vi "Auto_Inspection Station Main.vi"(8 "站別":refnum<vi>, 9 "站別":i32, 10 "ActRef":refnum<vi>, 11 "Station Action.lvclass":refnum<class "Station Action.lvclass">) -> ()   [LabVIEW 2019]
uses:
  Station Class/Station Action.lvclass
  Ctrl/Station Action.ctl
  Ctrl/Auto Inspection Data Name.ctl
  FlowCtrl Class/BarcodeScan/Ctl/Board Scan IO.ctl
  FlowCtrl Class/Ctrl/Auto Inspection_IN Name2.ctl
  Ctrl/ModbusCmd.ctl
  Ctrl/S2 Station IO.ctl
  FlowCtrl Class/Laser Detect/Ctl/S11 Station IO.ctl
  Function/Main UI/Glb/Main_UI Gb.vi
  Global/Process Global.vi
  Ctrl/Auto Inspection Main UI Ref.ctl
  LLB/Commonly VI.lvlib
  Ctrl/Auto Inspection Station Name2.ctl
  LLB/Commonly VI/Main Glb.vi
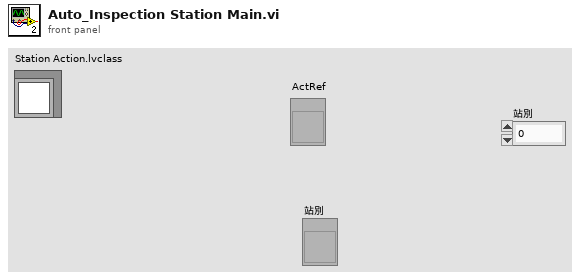
[diagram p1: front panel]
types:
  T1 = typedef "Station Action.ctl" = enum16{"Wait Item In", "Dectect Action", "ImformOut"}
  T2 = cluster{"AutoRunFlg":refnum<vi>, "Action Finish Flg":refnum<vi>, "Remaining Action":refnum<vi>, "Btn_AutoRun":refnum<vi>, "Manual Flg":refnum<vi>, "Sub Process Error":refnum<vi>}
  T3 = typedef "Auto Inspection Data Name.ctl" = enum16{"LocalRun", "ItemSN(TimeCode)", "CurrentAction", "Error", "Data", "OKNG", "電壓值", "電壓值判斷", "電流值", "電流值判斷", "Laser1 Data", "Laser2 Data", "Laser OKNG", "StationNO"}
  T4 = cluster{"starting address":u16, "number of inputs":u16, "Sat Coils":bool[], "Holding Registers":u16[]}
  T5 = typedef "ModbusCmd.ctl" = enum16{"Connect", "Disconnect", "Init", "Fetch Basic Objects", "Fetch Input Refisters", "Fetch Discrete Inputs", "Set Coils", "Set Holding Registers", "Write Single Holding", "Exit"}
  T6 = typedef "Auto Inspection_IN Name2.ctl" = enum16{"S0 Station", "S1 Barcode ", "S2 Tool Format", "S3 Tool Prpgram", "S4 Tool Sacn", "S11 Laser Detect", "S8 Vision AI"}
  T7 = typedef "Board Scan IO.ctl" = enum16{"S1 Barcode Scan", "回給PLC完成讀取訊號", "S1 載盤條碼比對NG", "S1PLC 條碼可讀取訊號", "S1備用_04", "S1備用_05", "S1備用_06", "S1備用_07", "S1備用_08", "S1 發送條碼完成"}
  T8 = typedef "S2 Station IO.ctl" = enum16{"S2站PC動作中_20", "電流量測完成產品OK_21", "電流量測完成產品NG_22", "S2站Format 執行_23", "S2 Format OK_24", "S2 Format NG_25", "S2站燒入執行_26", "S2站燒入OK_27", "S2站燒入NG_28", "S2站動作完成_29", "S3 PC動作中_30", "S3 Format 此站執行_31", "S3 Format OK_32", "S3 Format NG_33", "S3 燒入程式 此站執行_34", "S3 燒入程式 OK_35", "S3 燒入程式 NG_36", "S3 備用_37", "S3 備用_38", "S3 動作完成_39", "S4 PC動作中_40", "S4 量測完成 產品正常_41", "S4 量測完成 產品NG_42", "S4 Format 此站執行_43", "S4 Format OK_44", "S4 Format NG_45", "S4 燒入 此站不執行_46", "S4 燒入程式 OK_47", "S4 燒入程式 NG_48", "S4 藍芽Scan OK_49", "S4 藍芽Scan NG_50", "S4 動作完成_51", "給PLC要量電流訊號", "給PLC要量電壓訊號"}
  T9 = typedef "S11 Station IO.ctl" = enum16{"S11雷射測量動作中", "S11雷射測點1完成", "S11雷射測點2完成", "S11雷測測量OK", "S11雷測測量NG", "S11雷測測量重測", "S11備用_6", "S11備用_7", "S11備用_8", "S11雷射測高完成"}
  T10 = typedef "Auto Inspection Station Name2.ctl" = enum16{"S1Barcode", "S2Measure", "S3Measure", "S4Measure", "S5Measure", "S11_LaserCheck", "S8_Vision AI"}
  T11 = typedef "Auto Inspection Main UI Ref.ctl" = cluster{"LineScan arrive":refnum<vi>, "LineScanfinish":refnum<vi>, "AI arrive":refnum<vi>, "AI finish":refnum<vi>, "NG Pick arrive":refnum<vi>, "NG Pick finish":refnum<vi>}
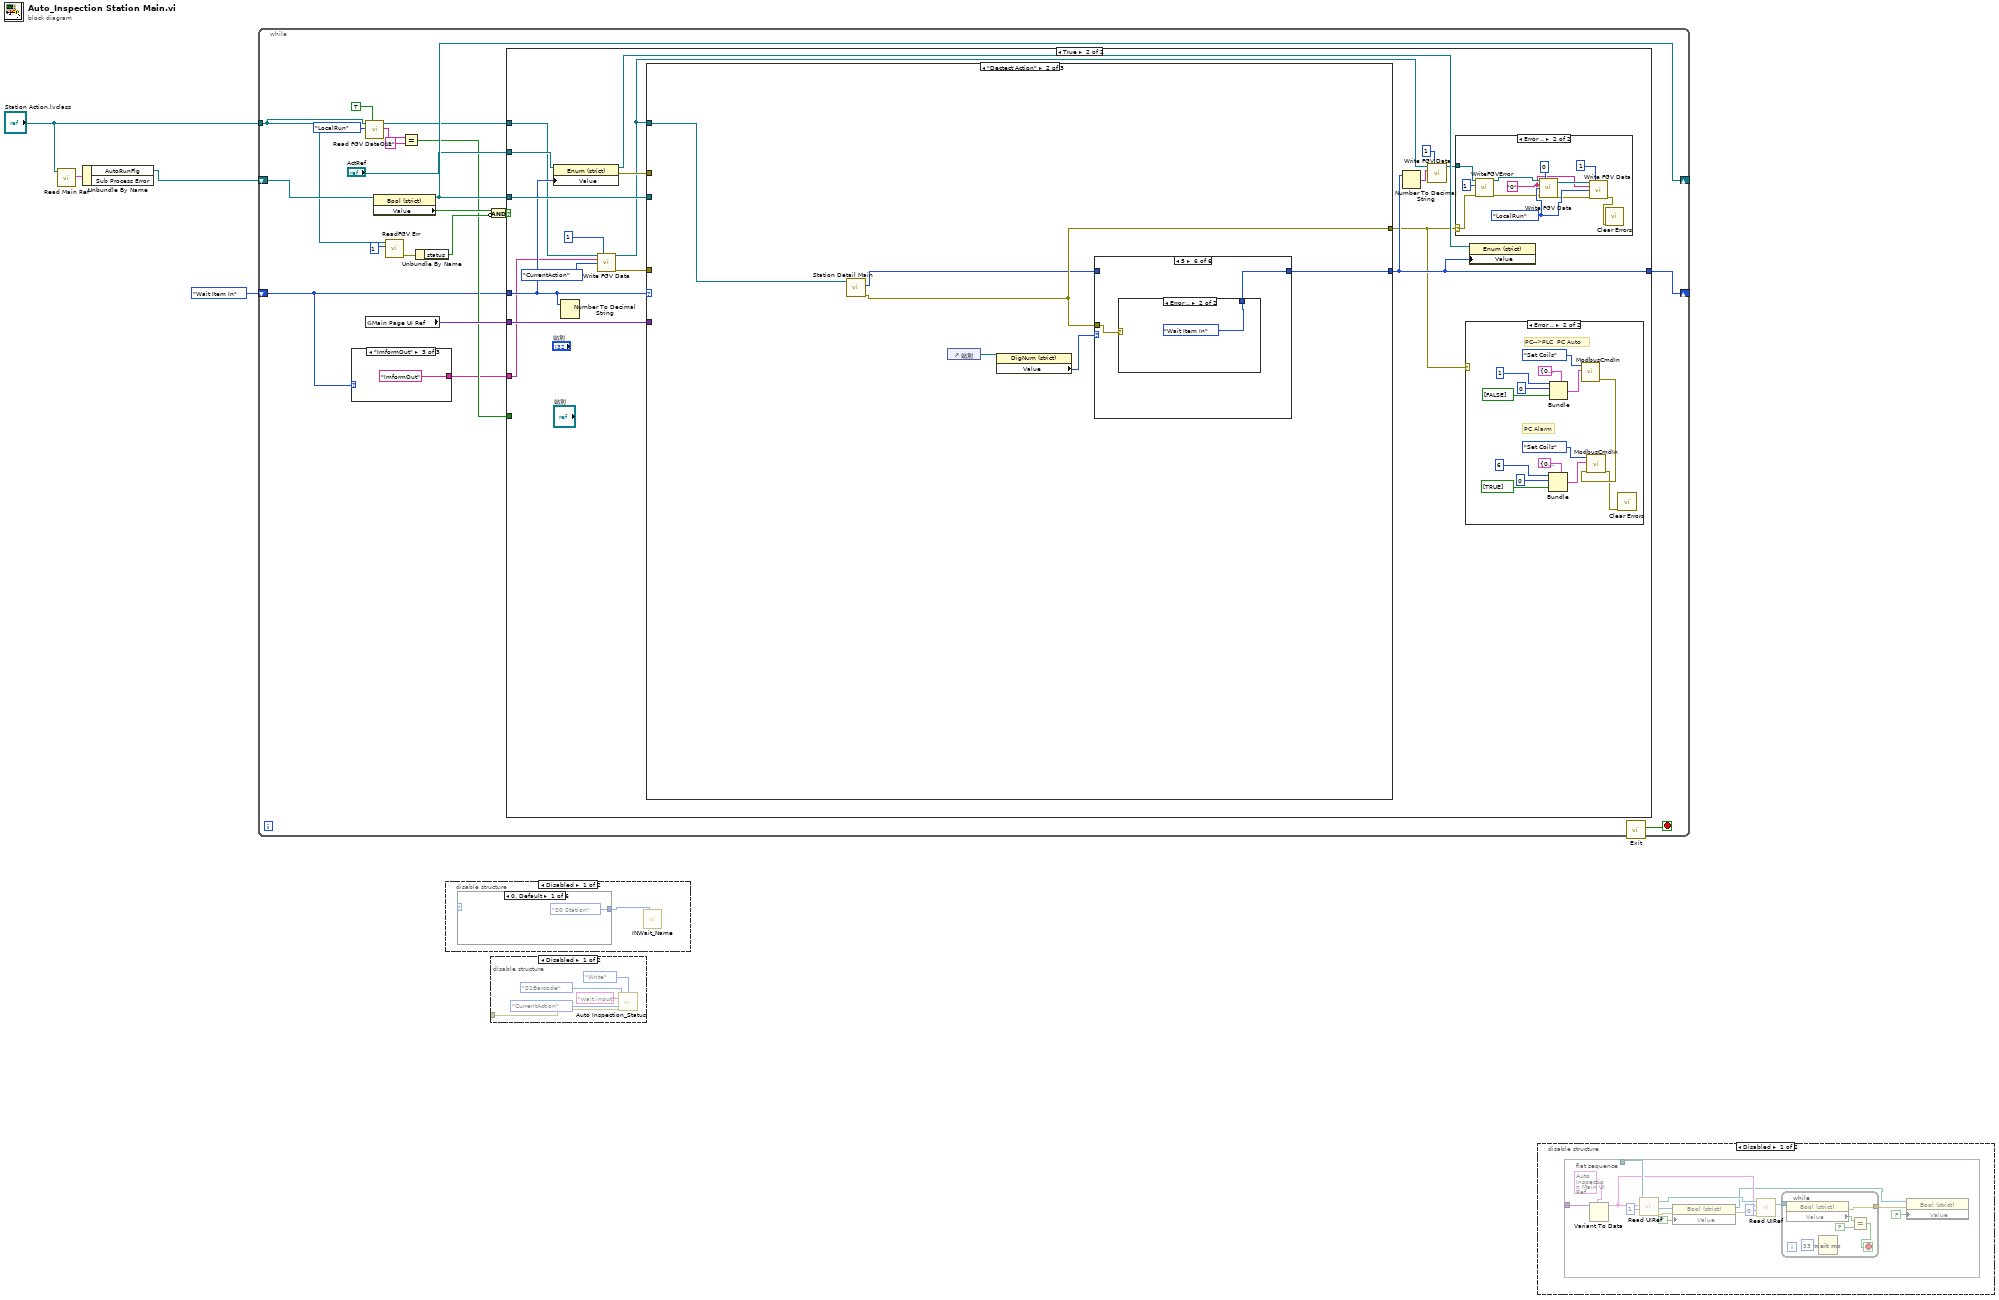
[diagram p0: block diagram]
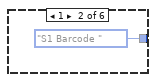
[diagram p2: hidden frame]
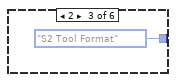
[diagram p3: hidden frame]
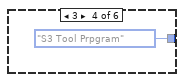
[diagram p4: hidden frame]
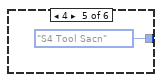
[diagram p5: hidden frame]
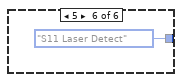
[diagram p6: hidden frame]
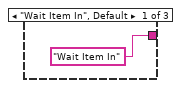
[diagram p10: hidden frame]
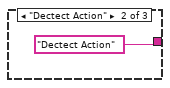
[diagram p11: hidden frame]
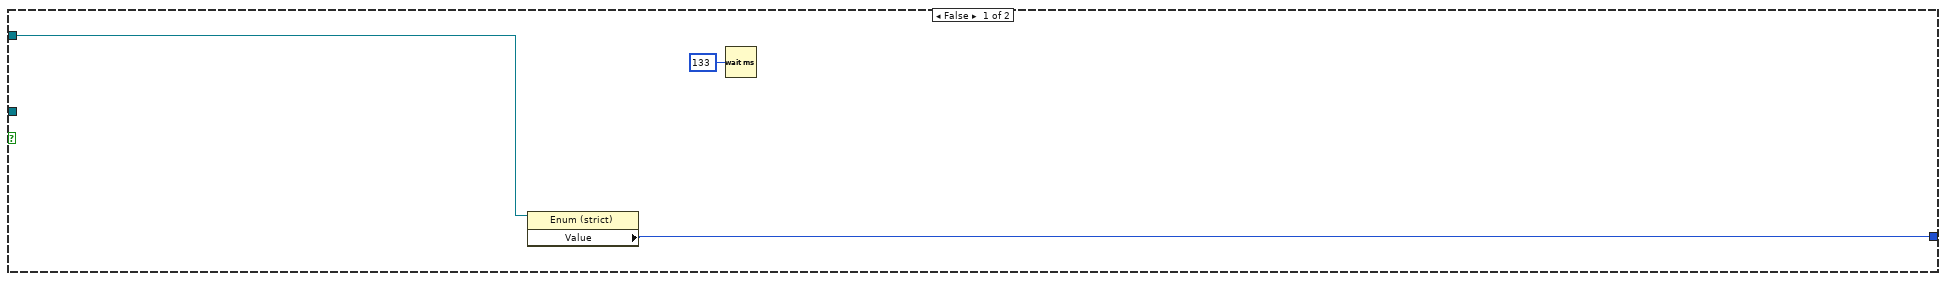
[diagram p12: hidden frame]
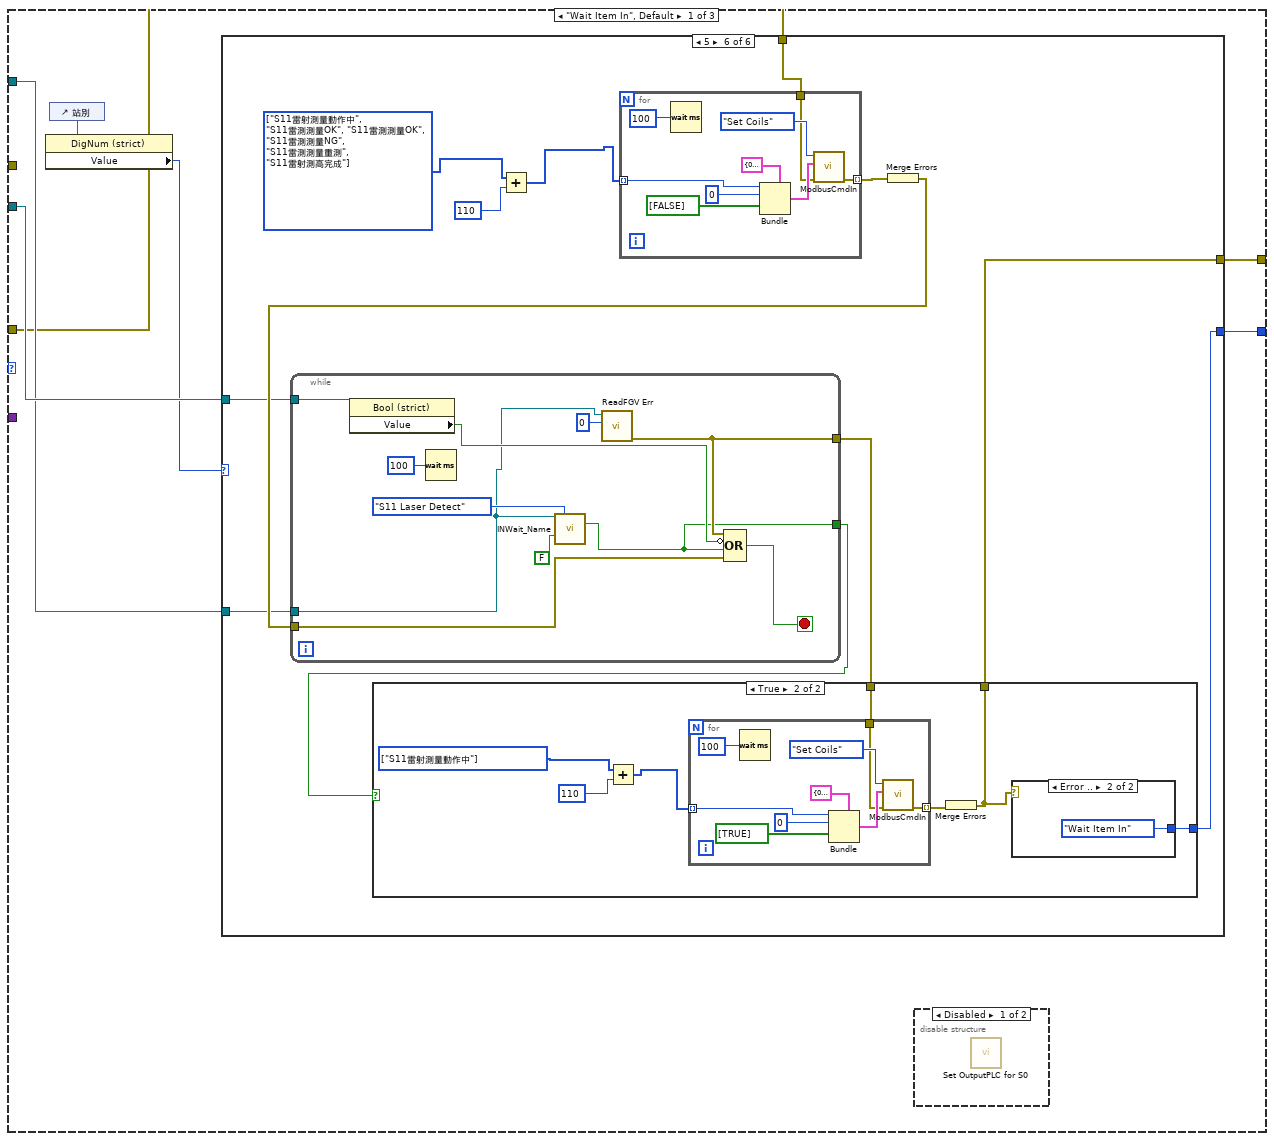
[diagram p15: hidden frame]
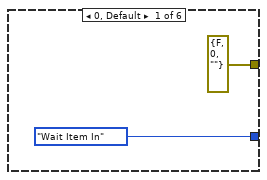
[diagram p17: hidden frame]
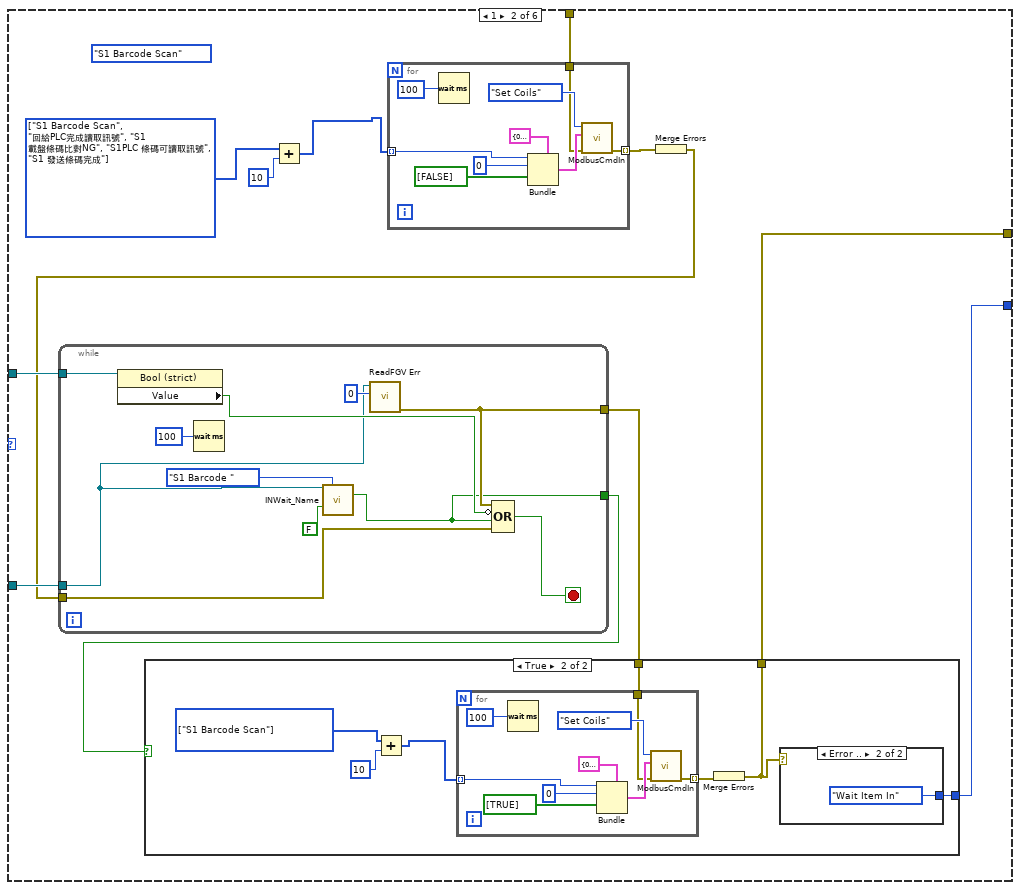
[diagram p18: hidden frame]
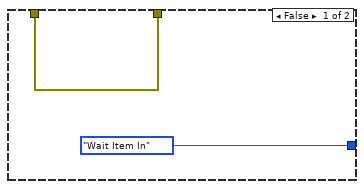
[diagram p19: hidden frame]
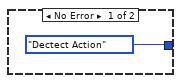
[diagram p20: hidden frame]
diagram:
  n1 = call-dynamic "Read Main Ref.vi"("Main Process Class in"="Station Action.lvclass") -> ("Main Ref"=w3:T2)  [unwired: 8 in, 2 out]
  n2 = Unbundle By Name(w3) -> ("AutoRunFlg"=w1:refnum<vi>)  [unwired: 1 out]
  n3 = while {
    shift-right: [w20] -> _
    shift-left: Station_Action."Wait Item In" -> [w6]
    tunnel: "Station Action.lvclass" -> [w8]
    shift-right: [w18] -> _
    shift-left: w1 -> [w23]
    stop <- w19 stop-if-true
    n4 = case shown="\"ImformOut\"" w6 {
      tunnel: ["Wait Item In" "Dectect Action" "ImformOut"] -> w5
      frame "Wait Item In", Default {
      }
      frame "Dectect Action" {
      }
      frame "ImformOut" {
      }
    }
    n5 = call-dynamic "Read FGV DataOut.vi"("TSt/FConveyor"=TRUE, "Data"=Auto_Inspection_Data_Name."LocalRun", "Station Action in"=w8) -> ("DataOut"=w11:string, "Station Action out"=w14:refnum<class "Station Action.lvclass">)  [unwired: 6 in, 1 out]
    n6 = global read "Main_UI Gb.vi" "Main Page UI Ref"() -> (w21:variant)
    n7 = property class="Bool (strict)"(reference=w23) -> (reference out=w18:refnum<vi>, "Value"=w24:bool)  [unwired: 1 in, 1 out]
    n8 = call-dynamic "ReadFGV Err.vi"("0Cv/1ST"=1, "Station Action in"=w8) -> ("error out"=w16:errorcluster)  [unwired: 8 in, 1 out]
    n9 = Equal?(x=w11, y="1") -> (x = y?=w7:bool)
    n10 = Unbundle By Name(w16) -> ("status"=w15:bool)
    n11 = Compound Arithmetic op=AND(w24, invert w15) -> (w22:bool)
    n12 = case shown="True" w22 {
      tunnel: w18 -> [_ w46]
      tunnel: w6 -> [_ w39]
      tunnel: w21 -> [_ w47]
      tunnel: w14 -> [_ w32]
      tunnel: [w29 w36] -> w20
      tunnel: "ActRef" -> [w30 w45]
      tunnel: w7 -> [_ _]
      tunnel: w5 -> [_ w31]
      frame False {
        n13 = property class="Enum (strict)"(reference=w30) -> ("Value"=w29:T1)  [unwired: 1 in, 2 out]
        n14 = Wait (ms)(milliseconds to wait=u32 133) -> ()  [unwired: 1 out]
      }
      frame True {
        n15 = property class="Enum (strict)"(reference=w45, "Value"=w39) -> (reference out=w44:refnum<vi>, error out=w43:errorcluster)  [unwired: 1 in]
        n16 = Number To Decimal String(number=w39) -> ()  [unwired: 1 in, 1 out]
        n17 = call-dynamic "Write FGV Data.vi"("Station Action in"=w32, "0Cv/1St"=1, "DataIn"=w31, "Data"=Auto_Inspection_Data_Name."CurrentAction") -> ("Station Action out"=w35:refnum<class "Station Action.lvclass">, "error out"=w40:errorcluster)  [unwired: 10 in]
        n18 = case shown="\"Dectect Action\"" w39 {
          tunnel: w47 -> [_ _ _]
          tunnel: w35 -> [w79 w352 w380]
          tunnel: w46 -> [w80 _ w379]
          tunnel: [w75 w350 w375] -> w36
          tunnel: w43 -> [_ _ _]
          tunnel: [w78 w351 w376] -> w33
          tunnel: w40 -> [w74 _ w378]
          frame "Wait Item In", Default {
            n19 = control-ref of="站別"() -> (w77:refnum<vi>)
            n20 = property class="DigNum (strict)"(reference=w77) -> ("Value"=w76:i32)  [unwired: 1 in, 2 out]
            n21 = case shown="5" w76 {
              tunnel: w80 -> [_ w94 w142 w195 w247 w298]
              tunnel: w79 -> [_ w93 w143 w194 w246 w300]
              tunnel: [errorcluster {"status"=FALSE, "code"=0, "source"=""} ("error IO") w92 w135 w197 w243 w299] -> w78
              tunnel: w74 -> [_ w91 _ w190 w248 w301]
              tunnel: [Station_Action."Wait Item In" w87 w144 w196 w245 w296] -> w75
              frame 0, Default {
              }
              frame 1 {
                (unwired) Board_Scan_IO."S1 Barcode Scan" ("Enum")
                w85 = T7[] [enum."S1 Barcode Scan", enum."回給PLC完成讀取訊號", enum."S1 載盤條碼比對NG", enum."S1PLC 條碼可讀取訊號", enum."S1 發送條碼完成"] items=["S1 Barcode Scan", "回給PLC完成讀取訊號", "S1 載盤條碼比對NG", "S1PLC 條碼可讀取訊號", "S1備用_04", "S1備用_05", "S1備用_06", "S1備用_07", "S1備用_08", "S1 發送條碼完成"]
                n22 = Add(x=w85, y=10) -> (x+y=w84:i32[])
                n23 = for {
                  tunnel: [w128] -> w90 mode=indexing
                  tunnel: w84 -> [w127] mode=indexing
                  tunnel: w91 -> [w126]
                  n24 = Wait (ms)(milliseconds to wait=100) -> ()  [unwired: 1 out]
                  n25 = Bundle(cluster=T4 {"starting address"=0, "number of inputs"=0, "Sat Coils"=[], "Holding Registers"=[]} ("data"), "starting address"=w127, "number of inputs"=u16 0, "Sat Coils"=bool[] [FALSE]) -> (w131:T4)  [unwired: 1 in]
                  n26 = call "ModbusCmdIn.vi"("error in (no error)"=w126, "data"=w131, "Enum"=ModbusCmd."Set Coils") -> ("error out"=w128:errorcluster)  [unwired: 8 in]
                }
                n27 = Merge Errors(w90) -> (w89:errorcluster)
                n28 = while {
                  tunnel: w94 -> [w125]
                  tunnel: w93 -> [w119]
                  tunnel: [w120] -> w88
                  tunnel: w89 -> [w117]
                  tunnel: [w116] -> w83
                  stop <- w124 stop-if-true
                  n29 = property class="Bool (strict)"(reference=w125) -> ("Value"=w122:bool)  [unwired: 1 in, 2 out]
                  n30 = Wait (ms)(milliseconds to wait=u32 100) -> ()  [unwired: 1 out]
                  n31 = call "INWait_Name.vi"("FlowCtrl in"=w119, "Input2"=Auto_Inspection_IN_Name2."S1 Barcode ", "Wait?"=FALSE) -> ("StatusOut"=w116:bool)  [unwired: 9 in, 3 out]
                  n32 = call-dynamic "ReadFGV Err.vi"("0Cv/1ST"=0, "Station Action in"=w119) -> ("error out"=w120:errorcluster)  [unwired: 8 in, 1 out]
                  n33 = Compound Arithmetic op=OR(w120, invert w122, w116, w117) -> (w124:bool)
                }
                n34 = case shown="True" w83 {
                  tunnel: [w96 w97] -> w92
                  tunnel: w88 -> [w96 w103]
                  tunnel: [Station_Action."Wait Item In" w100] -> w87
                  frame False {
                  }
                  frame True {
                    w99 = T7[] [enum."S1 Barcode Scan"] items=["S1 Barcode Scan", "回給PLC完成讀取訊號", "S1 載盤條碼比對NG", "S1PLC 條碼可讀取訊號", "S1備用_04", "S1備用_05", "S1備用_06", "S1備用_07", "S1備用_08", "S1 發送條碼完成"]
                    n35 = Add(x=w99, y=10) -> (x+y=w102:i32[])
                    n36 = for {
                      tunnel: [w108] -> w101 mode=indexing
                      tunnel: w102 -> [w107] mode=indexing
                      tunnel: w103 -> [w106]
                      n37 = Wait (ms)(milliseconds to wait=100) -> ()  [unwired: 1 out]
                      n38 = Bundle(cluster=T4 {"starting address"=0, "number of inputs"=0, "Sat Coils"=[], "Holding Registers"=[]} ("data"), "starting address"=w107, "number of inputs"=u16 0, "Sat Coils"=bool[] [TRUE]) -> (w111:T4)  [unwired: 1 in]
                      n39 = call "ModbusCmdIn.vi"("error in (no error)"=w106, "data"=w111, "Enum"=ModbusCmd."Set Coils") -> ("error out"=w108:errorcluster)  [unwired: 8 in]
                    }
                    n40 = Merge Errors(w101) -> (w97:errorcluster)
                    n41 = case shown="Error .." w97 {
                      tunnel: [Station_Action."Dectect Action" Station_Action."Wait Item In"] -> w100
                      frame No Error {
                      }
                      frame Error {
                      }
                    }
                  }
                }
              }
              frame 2 {
                w140 = T8[] [enum."S2站PC動作中_20", enum."電流量測完成產品OK_21", enum."電流量測完成產品NG_22", enum."S2 Format OK_24", enum."S2 Format NG_25", enum."S2站燒入OK_27", enum."S2站燒入NG_28", enum."S2站動作完成_29"] items=["S2站PC動作中_20", "電流量測完成產品OK_21", "電流量測完成產品NG_22", "S2站Format 執行_23", "S2 Format OK_24", "S2 Format NG_25", "S2站燒入執行_26", "S2站燒入OK_27", "S2站燒入NG_28", "S2站動作完成_29", "S3 PC動作中_30", "S3 Format 此站執行_31", "S3 Format OK_32", "S3 Format NG_33", "S3 燒入程式 此站執行_34", "S3 燒入程式 OK_35", "S3 燒入程式 NG_36", "S3 備用_37", "S3 備用_38", "S3 動作完成_39", "S4 PC動作中_40", "S4 量測完成 產品正常_41", "S4 量測完成 產品NG_42", "S4 Format 此站執行_43", "S4 Format OK_44", "S4 Format NG_45", "S4 燒入 此站不執行_46", "S4 燒入程式 OK_47", "S4 燒入程式 NG_48", "S4 藍芽Scan OK_49", "S4 藍芽Scan NG_50", "S4 動作完成_51", "給PLC要量電流訊號", "給PLC要量電壓訊號"]
                n42 = Add(x=w140, y=20) -> (x+y=w139:i32[])
                n43 = for {
                  tunnel: [w182] -> w145 mode=indexing
                  tunnel: w139 -> [w181] mode=indexing
                  n44 = Wait (ms)(milliseconds to wait=100) -> ()  [unwired: 1 out]
                  n45 = Bundle(cluster=T4 {"starting address"=0, "number of inputs"=0, "Sat Coils"=[], "Holding Registers"=[]} ("data"), "starting address"=w181, "number of inputs"=u16 0, "Sat Coils"=bool[] [FALSE]) -> (w185:T4)  [unwired: 1 in]
                  n46 = call "ModbusCmdIn.vi"("data"=w185, "Enum"=ModbusCmd."Set Coils") -> ("error out"=w182:errorcluster)  [unwired: 9 in]
                }
                n47 = Merge Errors(w145) -> (w146:errorcluster)
                n48 = while {
                  tunnel: w143 -> [w175]
                  tunnel: [w176] -> w147
                  tunnel: w146 -> [w170]
                  tunnel: [w173] -> w138
                  tunnel: w142 -> [w171]
                  tunnel: [w170] -> w136
                  stop <- w180 stop-if-true
                  n49 = property class="Bool (strict)"(reference=w171) -> ("Value"=w178:bool)  [unwired: 1 in, 2 out]
                  n50 = Wait (ms)(milliseconds to wait=u32 100) -> ()  [unwired: 1 out]
                  n51 = call "INWait_Name.vi"("FlowCtrl in"=w175, "Input2"=Auto_Inspection_IN_Name2."S2 Tool Format", "Wait?"=FALSE) -> ("StatusOut"=w173:bool)  [unwired: 9 in, 3 out]
                  n52 = call-dynamic "ReadFGV Err.vi"("0Cv/1ST"=0, "Station Action in"=w175) -> ("error out"=w176:errorcluster)  [unwired: 8 in, 1 out]
                  n53 = Compound Arithmetic op=OR(w176, invert w178, w173, w170) -> (w180:bool)
                }
                n54 = case shown="True" w138 {
                  tunnel: w147 -> [w149 w157]
                  tunnel: [w149 w152] -> w137
                  tunnel: [Station_Action."Wait Item In" w156] -> w144
                  frame False {
                  }
                  frame True {
                    w155 = T8[] [enum."S2站PC動作中_20"] items=["S2站PC動作中_20", "電流量測完成產品OK_21", "電流量測完成產品NG_22", "S2站Format 執行_23", "S2 Format OK_24", "S2 Format NG_25", "S2站燒入執行_26", "S2站燒入OK_27", "S2站燒入NG_28", "S2站動作完成_29", "S3 PC動作中_30", "S3 Format 此站執行_31", "S3 Format OK_32", "S3 Format NG_33", "S3 燒入程式 此站執行_34", "S3 燒入程式 OK_35", "S3 燒入程式 NG_36", "S3 備用_37", "S3 備用_38", "S3 動作完成_39", "S4 PC動作中_40", "S4 量測完成 產品正常_41", "S4 量測完成 產品NG_42", "S4 Format 此站執行_43", "S4 Format OK_44", "S4 Format NG_45", "S4 燒入 此站不執行_46", "S4 燒入程式 OK_47", "S4 燒入程式 NG_48", "S4 藍芽Scan OK_49", "S4 藍芽Scan NG_50", "S4 動作完成_51", "給PLC要量電流訊號", "給PLC要量電壓訊號"]
                    n55 = global write "Process Global.vi" "S2 NG"(FALSE) -> ()
                    n56 = global write "Process Global.vi" "S2 OK"(FALSE) -> ()
                    n57 = Add(x=w155, y=20) -> (x+y=w153:i32[])
                    n58 = for {
                      tunnel: [w163] -> w158 mode=indexing
                      tunnel: w153 -> [w162] mode=indexing
                      tunnel: w157 -> [w161]
                      n59 = Wait (ms)(milliseconds to wait=100) -> ()  [unwired: 1 out]
                      n60 = Bundle(cluster=T4 {"starting address"=0, "number of inputs"=0, "Sat Coils"=[], "Holding Registers"=[]} ("data"), "starting address"=w162, "number of inputs"=u16 0, "Sat Coils"=bool[] [TRUE]) -> (w166:T4)  [unwired: 1 in]
                      n61 = call "ModbusCmdIn.vi"("error in (no error)"=w161, "data"=w166, "Enum"=ModbusCmd."Set Coils") -> ("error out"=w163:errorcluster)  [unwired: 8 in]
                    }
                    n62 = Merge Errors(w158) -> (w152:errorcluster)
                    n63 = case shown="Error .." w152 {
                      tunnel: [Station_Action."Dectect Action" Station_Action."Wait Item In"] -> w156
                      frame No Error {
                      }
                      frame Error {
                      }
                    }
                  }
                }
                n64 = Merge Errors(w136, w137) -> (w135:errorcluster)
              }
              frame 3 {
                w193 = T8[] [enum."S3 PC動作中_30", enum."S3 Format OK_32", enum."S3 Format NG_33", enum."S3 燒入程式 OK_35", enum."S3 燒入程式 NG_36", enum."S3 動作完成_39"] items=["S2站PC動作中_20", "電流量測完成產品OK_21", "電流量測完成產品NG_22", "S2站Format 執行_23", "S2 Format OK_24", "S2 Format NG_25", "S2站燒入執行_26", "S2站燒入OK_27", "S2站燒入NG_28", "S2站動作完成_29", "S3 PC動作中_30", "S3 Format 此站執行_31", "S3 Format OK_32", "S3 Format NG_33", "S3 燒入程式 此站執行_34", "S3 燒入程式 OK_35", "S3 燒入程式 NG_36", "S3 備用_37", "S3 備用_38", "S3 動作完成_39", "S4 PC動作中_40", "S4 量測完成 產品正常_41", "S4 量測完成 產品NG_42", "S4 Format 此站執行_43", "S4 Format OK_44", "S4 Format NG_45", "S4 燒入 此站不執行_46", "S4 燒入程式 OK_47", "S4 燒入程式 NG_48", "S4 藍芽Scan OK_49", "S4 藍芽Scan NG_50", "S4 動作完成_51", "給PLC要量電流訊號", "給PLC要量電壓訊號"]
                n65 = Add(x=w193, y=20) -> (x+y=w191:i32[])
                n66 = for {
                  tunnel: [w235] -> w198 mode=indexing
                  tunnel: w191 -> [w234] mode=indexing
                  tunnel: w190 -> [w233]
                  n67 = Wait (ms)(milliseconds to wait=100) -> ()  [unwired: 1 out]
                  n68 = Bundle(cluster=T4 {"starting address"=0, "number of inputs"=0, "Sat Coils"=[], "Holding Registers"=[]} ("data"), "starting address"=w234, "number of inputs"=u16 0, "Sat Coils"=bool[] [FALSE]) -> (w238:T4)  [unwired: 1 in]
                  n69 = call "ModbusCmdIn.vi"("error in (no error)"=w233, "data"=w238, "Enum"=ModbusCmd."Set Coils") -> ("error out"=w235:errorcluster)  [unwired: 8 in]
                }
                n70 = Merge Errors(w198) -> (w199:errorcluster)
                n71 = while {
                  tunnel: w195 -> [w232]
                  tunnel: w194 -> [w226]
                  tunnel: [w227] -> w200
                  tunnel: w199 -> [w224]
                  tunnel: [w223] -> w189
                  stop <- w231 stop-if-true
                  n72 = property class="Bool (strict)"(reference=w232) -> ("Value"=w229:bool)  [unwired: 1 in, 2 out]
                  n73 = Wait (ms)(milliseconds to wait=u32 100) -> ()  [unwired: 1 out]
                  n74 = call "INWait_Name.vi"("FlowCtrl in"=w226, "Input2"=Auto_Inspection_IN_Name2."S3 Tool Prpgram", "Wait?"=FALSE) -> ("StatusOut"=w223:bool)  [unwired: 9 in, 3 out]
                  n75 = call-dynamic "ReadFGV Err.vi"("0Cv/1ST"=0, "Station Action in"=w226) -> ("error out"=w227:errorcluster)  [unwired: 8 in, 1 out]
                  n76 = Compound Arithmetic op=OR(w227, invert w229, w223, w224) -> (w231:bool)
                }
                n77 = case shown="True" w189 {
                  tunnel: w200 -> [w202 w209]
                  tunnel: [w202 w204] -> w197
                  tunnel: [Station_Action."Wait Item In" w208] -> w196
                  frame False {
                  }
                  frame True {
                    w203 = FALSE ("S3 NG")
                    w206 = T8[] [enum."S3 PC動作中_30"] items=["S2站PC動作中_20", "電流量測完成產品OK_21", "電流量測完成產品NG_22", "S2站Format 執行_23", "S2 Format OK_24", "S2 Format NG_25", "S2站燒入執行_26", "S2站燒入OK_27", "S2站燒入NG_28", "S2站動作完成_29", "S3 PC動作中_30", "S3 Format 此站執行_31", "S3 Format OK_32", "S3 Format NG_33", "S3 燒入程式 此站執行_34", "S3 燒入程式 OK_35", "S3 燒入程式 NG_36", "S3 備用_37", "S3 備用_38", "S3 動作完成_39", "S4 PC動作中_40", "S4 量測完成 產品正常_41", "S4 量測完成 產品NG_42", "S4 Format 此站執行_43", "S4 Format OK_44", "S4 Format NG_45", "S4 燒入 此站不執行_46", "S4 燒入程式 OK_47", "S4 燒入程式 NG_48", "S4 藍芽Scan OK_49", "S4 藍芽Scan NG_50", "S4 動作完成_51", "給PLC要量電流訊號", "給PLC要量電壓訊號"]
                    n78 = global write "Process Global.vi" "S3 NG"(w203) -> ()
                    n79 = global write "Process Global.vi" "S3 OK"(w203) -> ()
                    n80 = Add(x=w206, y=20) -> (x+y=w205:i32[])
                    n81 = for {
                      tunnel: [w215] -> w210 mode=indexing
                      tunnel: w205 -> [w214] mode=indexing
                      tunnel: w209 -> [w213]
                      n82 = Wait (ms)(milliseconds to wait=100) -> ()  [unwired: 1 out]
                      n83 = Bundle(cluster=T4 {"starting address"=0, "number of inputs"=0, "Sat Coils"=[], "Holding Registers"=[]} ("data"), "starting address"=w214, "number of inputs"=u16 0, "Sat Coils"=bool[] [TRUE]) -> (w218:T4)  [unwired: 1 in]
                      n84 = call "ModbusCmdIn.vi"("error in (no error)"=w213, "data"=w218, "Enum"=ModbusCmd."Set Coils") -> ("error out"=w215:errorcluster)  [unwired: 8 in]
                    }
                    n85 = Merge Errors(w210) -> (w204:errorcluster)
                    n86 = case shown="Error .." w204 {
                      tunnel: [Station_Action."Dectect Action" Station_Action."Wait Item In"] -> w208
                      frame No Error {
                      }
                      frame Error {
                      }
                    }
                  }
                }
              }
              frame 4 {
                w244 = T8[] [enum."S4 PC動作中_40", enum."S4 量測完成 產品正常_41", enum."S4 量測完成 產品NG_42", enum."S4 Format OK_44", enum."S4 Format NG_45", enum."S4 燒入程式 OK_47", enum."S4 燒入程式 NG_48", enum."S4 藍芽Scan OK_49", enum."S4 藍芽Scan NG_50", enum."S4 動作完成_51"] items=["S2站PC動作中_20", "電流量測完成產品OK_21", "電流量測完成產品NG_22", "S2站Format 執行_23", "S2 Format OK_24", "S2 Format NG_25", "S2站燒入執行_26", "S2站燒入OK_27", "S2站燒入NG_28", "S2站動作完成_29", "S3 PC動作中_30", "S3 Format 此站執行_31", "S3 Format OK_32", "S3 Format NG_33", "S3 燒入程式 此站執行_34", "S3 燒入程式 OK_35", "S3 燒入程式 NG_36", "S3 備用_37", "S3 備用_38", "S3 動作完成_39", "S4 PC動作中_40", "S4 量測完成 產品正常_41", "S4 量測完成 產品NG_42", "S4 Format 此站執行_43", "S4 Format OK_44", "S4 Format NG_45", "S4 燒入 此站不執行_46", "S4 燒入程式 OK_47", "S4 燒入程式 NG_48", "S4 藍芽Scan OK_49", "S4 藍芽Scan NG_50", "S4 動作完成_51", "給PLC要量電流訊號", "給PLC要量電壓訊號"]
                n87 = Add(x=w244, y=20) -> (x+y=w253:i32[])
                n88 = for {
                  tunnel: [w288] -> w249 mode=indexing
                  tunnel: w253 -> [w287] mode=indexing
                  tunnel: w248 -> [w286]
                  n89 = Wait (ms)(milliseconds to wait=100) -> ()  [unwired: 1 out]
                  n90 = Bundle(cluster=T4 {"starting address"=0, "number of inputs"=0, "Sat Coils"=[], "Holding Registers"=[]} ("data"), "starting address"=w287, "number of inputs"=u16 0, "Sat Coils"=bool[] [FALSE]) -> (w291:T4)  [unwired: 1 in]
                  n91 = call "ModbusCmdIn.vi"("error in (no error)"=w286, "data"=w291, "Enum"=ModbusCmd."Set Coils") -> ("error out"=w288:errorcluster)  [unwired: 8 in]
                }
                n92 = Merge Errors(w249) -> (w250:errorcluster)
                n93 = while {
                  tunnel: [w281] -> w251
                  tunnel: w250 -> [w279]
                  tunnel: [w278] -> w242
                  tunnel: w247 -> [w276]
                  tunnel: w246 -> [w275]
                  stop <- w285 stop-if-true
                  n94 = property class="Bool (strict)"(reference=w276) -> ("Value"=w283:bool)  [unwired: 1 in, 2 out]
                  n95 = Wait (ms)(milliseconds to wait=u32 100) -> ()  [unwired: 1 out]
                  n96 = call "INWait_Name.vi"("FlowCtrl in"=w275, "Input2"=Auto_Inspection_IN_Name2."S4 Tool Sacn", "Wait?"=FALSE) -> ("StatusOut"=w278:bool)  [unwired: 9 in, 3 out]
                  n97 = call-dynamic "ReadFGV Err.vi"("0Cv/1ST"=0, "Station Action in"=w275) -> ("error out"=w281:errorcluster)  [unwired: 8 in, 1 out]
                  n98 = Compound Arithmetic op=OR(w281, invert w283, w278, w279) -> (w285:bool)
                }
                n99 = case shown="True" w242 {
                  tunnel: w251 -> [w255 w260]
                  tunnel: [Station_Action."Wait Item In" w259] -> w245
                  tunnel: [w255 w257] -> w243
                  frame False {
                  }
                  frame True {
                    w256 = FALSE ("S4 NG")
                    w258 = T8[] [enum."S4 PC動作中_40"] items=["S2站PC動作中_20", "電流量測完成產品OK_21", "電流量測完成產品NG_22", "S2站Format 執行_23", "S2 Format OK_24", "S2 Format NG_25", "S2站燒入執行_26", "S2站燒入OK_27", "S2站燒入NG_28", "S2站動作完成_29", "S3 PC動作中_30", "S3 Format 此站執行_31", "S3 Format OK_32", "S3 Format NG_33", "S3 燒入程式 此站執行_34", "S3 燒入程式 OK_35", "S3 燒入程式 NG_36", "S3 備用_37", "S3 備用_38", "S3 動作完成_39", "S4 PC動作中_40", "S4 量測完成 產品正常_41", "S4 量測完成 產品NG_42", "S4 Format 此站執行_43", "S4 Format OK_44", "S4 Format NG_45", "S4 燒入 此站不執行_46", "S4 燒入程式 OK_47", "S4 燒入程式 NG_48", "S4 藍芽Scan OK_49", "S4 藍芽Scan NG_50", "S4 動作完成_51", "給PLC要量電流訊號", "給PLC要量電壓訊號"]
                    n100 = global write "Process Global.vi" "S4 NG"(w256) -> ()
                    n101 = global write "Process Global.vi" "S4 OK"(w256) -> ()
                    n102 = Add(x=w258, y=20) -> (x+y=w261:i32[])
                    n103 = for {
                      tunnel: [w268] -> w262 mode=indexing
                      tunnel: w261 -> [w267] mode=indexing
                      tunnel: w260 -> [w266]
                      n104 = Wait (ms)(milliseconds to wait=100) -> ()  [unwired: 1 out]
                      n105 = Bundle(cluster=T4 {"starting address"=0, "number of inputs"=0, "Sat Coils"=[], "Holding Registers"=[]} ("data"), "starting address"=w267, "number of inputs"=u16 0, "Sat Coils"=bool[] [TRUE]) -> (w271:T4)  [unwired: 1 in]
                      n106 = call "ModbusCmdIn.vi"("error in (no error)"=w266, "data"=w271, "Enum"=ModbusCmd."Set Coils") -> ("error out"=w268:errorcluster)  [unwired: 8 in]
                    }
                    n107 = Merge Errors(w262) -> (w257:errorcluster)
                    n108 = case shown="Error .." w257 {
                      tunnel: [Station_Action."Dectect Action" Station_Action."Wait Item In"] -> w259
                      frame No Error {
                      }
                      frame Error {
                      }
                    }
                  }
                }
              }
              frame 5 {
                w297 = T9[] [enum."S11雷射測量動作中", enum."S11雷測測量OK", enum."S11雷測測量OK", enum."S11雷測測量NG", enum."S11雷測測量重測", enum."S11雷射測高完成"] items=["S11雷射測量動作中", "S11雷射測點1完成", "S11雷射測點2完成", "S11雷測測量OK", "S11雷測測量NG", "S11雷測測量重測", "S11備用_6", "S11備用_7", "S11備用_8", "S11雷射測高完成"]
                n109 = Add(x=w297, y=110) -> (x+y=w306:i32[])
                n110 = for {
                  tunnel: [w340] -> w302 mode=indexing
                  tunnel: w306 -> [w339] mode=indexing
                  tunnel: w301 -> [w338]
                  n111 = Wait (ms)(milliseconds to wait=100) -> ()  [unwired: 1 out]
                  n112 = Bundle(cluster=T4 {"starting address"=0, "number of inputs"=0, "Sat Coils"=[], "Holding Registers"=[]} ("data"), "starting address"=w339, "number of inputs"=u16 0, "Sat Coils"=bool[] [FALSE]) -> (w343:T4)  [unwired: 1 in]
                  n113 = call "ModbusCmdIn.vi"("error in (no error)"=w338, "data"=w343, "Enum"=ModbusCmd."Set Coils") -> ("error out"=w340:errorcluster)  [unwired: 8 in]
                }
                n114 = Merge Errors(w302) -> (w303:errorcluster)
                n115 = while {
                  tunnel: [w333] -> w304
                  tunnel: w303 -> [w331]
                  tunnel: [w330] -> w295
                  tunnel: w300 -> [w327]
                  tunnel: w298 -> [w328]
                  stop <- w337 stop-if-true
                  n116 = property class="Bool (strict)"(reference=w328) -> ("Value"=w335:bool)  [unwired: 1 in, 2 out]
                  n117 = Wait (ms)(milliseconds to wait=u32 100) -> ()  [unwired: 1 out]
                  n118 = call "INWait_Name.vi"("FlowCtrl in"=w327, "Input2"=Auto_Inspection_IN_Name2."S11 Laser Detect", "Wait?"=FALSE) -> ("StatusOut"=w330:bool)  [unwired: 9 in, 3 out]
                  n119 = call-dynamic "ReadFGV Err.vi"("0Cv/1ST"=0, "Station Action in"=w327) -> ("error out"=w333:errorcluster)  [unwired: 8 in, 1 out]
                  n120 = Compound Arithmetic op=OR(w333, invert w335, w330, w331) -> (w337:bool)
                }
                n121 = case shown="True" w295 {
                  tunnel: w304 -> [w307 w312]
                  tunnel: [w307 w310] -> w299
                  tunnel: [Station_Action."Wait Item In" w309] -> w296
                  frame False {
                  }
                  frame True {
                    w311 = T9[] [enum."S11雷射測量動作中"] items=["S11雷射測量動作中", "S11雷射測點1完成", "S11雷射測點2完成", "S11雷測測量OK", "S11雷測測量NG", "S11雷測測量重測", "S11備用_6", "S11備用_7", "S11備用_8", "S11雷射測高完成"]
                    n122 = Add(x=w311, y=110) -> (x+y=w313:i32[])
                    n123 = for {
                      tunnel: [w320] -> w314 mode=indexing
                      tunnel: w313 -> [w319] mode=indexing
                      tunnel: w312 -> [w318]
                      n124 = Wait (ms)(milliseconds to wait=100) -> ()  [unwired: 1 out]
                      n125 = Bundle(cluster=T4 {"starting address"=0, "number of inputs"=0, "Sat Coils"=[], "Holding Registers"=[]} ("data"), "starting address"=w319, "number of inputs"=u16 0, "Sat Coils"=bool[] [TRUE]) -> (w323:T4)  [unwired: 1 in]
                      n126 = call "ModbusCmdIn.vi"("error in (no error)"=w318, "data"=w323, "Enum"=ModbusCmd."Set Coils") -> ("error out"=w320:errorcluster)  [unwired: 8 in]
                    }
                    n127 = Merge Errors(w314) -> (w310:errorcluster)
                    n128 = case shown="Error .." w310 {
                      tunnel: [Station_Action."Dectect Action" Station_Action."Wait Item In"] -> w309
                      frame No Error {
                      }
                      frame Error {
                      }
                    }
                  }
                }
              }
            }
            n129 = disable-structure shown="Disabled" {
              frame Disabled {
                n130 = call "Set OutputPLC for S0.vi"() -> ()  [unwired: 10 in, 1 out]
              }
              frame Enabled {
              }
            }
          }
          frame "Dectect Action" {
            n131 = call-dynamic "Station Detail Main.vi"("Station Action in"=w352) -> ("error out"=w351:errorcluster, "Station Out"=w347:T1)  [unwired: 8 in, 1 out]
            n132 = control-ref of="站別"() -> (w349:refnum<vi>)
            n133 = property class="DigNum (strict)"(reference=w349) -> ("Value"=w348:i32)  [unwired: 1 in, 2 out]
            n134 = case shown="5" w348 {
              tunnel: w351 -> [_ w355 w358 w362 w366 w370]
              tunnel: [w353 w354 w359 w363 w367 w371] -> w350
              tunnel: w347 -> [w353 _ _ _ _ _]
              frame 0, Default {
              }
              frame 1 {
                n135 = case shown="Error .." w355 {
                  tunnel: [Station_Action."ImformOut" ("Station Out") Station_Action."Wait Item In" ("Station Out")] -> w354
                  frame No Error {
                  }
                  frame Error {
                  }
                }
              }
              frame 2 {
                n136 = case shown="Error .." w358 {
                  tunnel: [Station_Action."ImformOut" ("Station Out") Station_Action."Wait Item In" ("Station Out")] -> w359
                  frame No Error {
                  }
                  frame Error {
                  }
                }
              }
              frame 3 {
                n137 = case shown="Error .." w362 {
                  tunnel: [Station_Action."ImformOut" ("Station Out") Station_Action."Wait Item In" ("Station Out")] -> w363
                  frame No Error {
                  }
                  frame Error {
                  }
                }
              }
              frame 4 {
                n138 = case shown="Error .." w366 {
                  tunnel: [Station_Action."ImformOut" ("Station Out") Station_Action."Wait Item In" ("Station Out")] -> w367
                  frame No Error {
                  }
                  frame Error {
                  }
                }
              }
              frame 5 {
                n139 = case shown="Error .." w370 {
                  tunnel: [Station_Action."ImformOut" ("Station Out") Station_Action."Wait Item In" ("Station Out")] -> w371
                  frame No Error {
                  }
                  frame Error {
                  }
                }
              }
            }
          }
          frame "ImformOut" {
            # "AutoRunFlg"
            n140 = control-ref of="站別"() -> (w377:refnum<vi>)
            n141 = property class="DigNum (strict)"(reference=w377) -> ("Value"=w374:i32)  [unwired: 1 in, 2 out]
            n142 = case shown="5" w374 {
              selector: w374 -> [_ _ _ w497 _ _]
              tunnel: w380 -> [_ w395 w442 w499 w555 w625]
              tunnel: w379 -> [_ w394 w441 w498 w554 w624]
              tunnel: w378 -> [_ w393 w445 w502 w556 w626]
              tunnel: w374 -> [_ _ _ _ _ _]
              tunnel: [errorcluster {"status"=FALSE, "code"=0, "source"=""} ("error IO") w386 w440 w495 w558 w622] -> w376
              tunnel: [Station_Action."Wait Item In" w385 w439 w496 w557 w623] -> w375
              frame 0, Default {
              }
              frame 1 {
                w384 = T7[] [enum."S1 Barcode Scan"] items=["S1 Barcode Scan", "回給PLC完成讀取訊號", "S1 載盤條碼比對NG", "S1PLC 條碼可讀取訊號", "S1備用_04", "S1備用_05", "S1備用_06", "S1備用_07", "S1備用_08", "S1 發送條碼完成"]
                n143 = Add(x=w384, y=10) -> (x+y=w392:i32[])
                n144 = for {
                  tunnel: [w401] -> w391 mode=indexing
                  tunnel: w393 -> [w400]
                  tunnel: w392 -> [w399] mode=indexing
                  tunnel: bool[] [FALSE] ("Sat Coils") -> [w398]
                  n145 = Wait (ms)(milliseconds to wait=100) -> ()  [unwired: 1 out]
                  n146 = Bundle(cluster=T4 {"starting address"=0, "number of inputs"=0, "Sat Coils"=[], "Holding Registers"=[]} ("data"), "starting address"=w399, "number of inputs"=u16 0, "Sat Coils"=w398) -> (w404:T4)  [unwired: 1 in]
                  n147 = call "ModbusCmdIn.vi"("error in (no error)"=w400, "data"=w404, "Enum"=ModbusCmd."Set Coils") -> ("error out"=w401:errorcluster)  [unwired: 8 in]
                }
                n148 = Merge Errors(w391) -> (w390:errorcluster)
                n149 = while {
                  tunnel: w395 -> [w437]
                  tunnel: w394 -> [w436]
                  tunnel: [w429] -> w389
                  tunnel: [w432] -> w388
                  tunnel: w390 -> [w426]
                  stop <- w433 stop-if-true
                  n150 = property class="Bool (strict)"(reference=w436) -> ("Value"=w435:bool)  [unwired: 1 in, 2 out]
                  n151 = Not(x=w435) -> (.not. x?=w434:bool)
                  n152 = call "INWait_Name.vi"("FlowCtrl in"=w437, "Input2"=Auto_Inspection_IN_Name2."S1 Barcode ", "Wait?"=FALSE, "error in (no error)"=w426) -> ("StatusOut"=w431:bool, "error out"=w432:errorcluster)  [unwired: 8 in, 2 out]
                  n153 = Equal?(x=FALSE, y=w431) -> (x = y?=w429:bool)
                  n154 = Compound Arithmetic op=OR(w426, w429, w434) -> (w433:bool)
                  n155 = Wait (ms)(milliseconds to wait=123) -> ()  [unwired: 1 out]
                }
                n156 = case shown="True" w389 {
                  tunnel: w388 -> [w407 w413]
                  tunnel: [w407 w410] -> w386
                  frame False {
                  }
                  frame True {
                    w409 = T7[] [enum."S1 Barcode Scan", enum."回給PLC完成讀取訊號", enum."S1 載盤條碼比對NG", enum."S1PLC 條碼可讀取訊號", enum."S1 發送條碼完成"] items=["S1 Barcode Scan", "回給PLC完成讀取訊號", "S1 載盤條碼比對NG", "S1PLC 條碼可讀取訊號", "S1備用_04", "S1備用_05", "S1備用_06", "S1備用_07", "S1備用_08", "S1 發送條碼完成"]
                    n157 = Add(x=w409, y=10) -> (x+y=w412:i32[])
                    n158 = for {
                      tunnel: w412 -> [w417] mode=indexing
                      tunnel: [w419] -> w414 mode=indexing
                      tunnel: w413 -> [w418]
                      n159 = Wait (ms)(milliseconds to wait=100) -> ()  [unwired: 1 out]
                      n160 = Bundle(cluster=T4 {"starting address"=0, "number of inputs"=0, "Sat Coils"=[], "Holding Registers"=[]} ("data"), "starting address"=w417, "number of inputs"=u16 0, "Sat Coils"=bool[] [FALSE]) -> (w422:T4)  [unwired: 1 in]
                      n161 = call "ModbusCmdIn.vi"("error in (no error)"=w418, "data"=w422, "Enum"=ModbusCmd."Set Coils") -> ("error out"=w419:errorcluster)  [unwired: 8 in]
                    }
                    n162 = Merge Errors(w414) -> (w411:errorcluster)
                    n163 = case shown="No Error" w411 {
                      selector: w411 -> [w415 w416]
                      tunnel: [w415 w416] -> w410
                      frame No Error {
                      }
                      frame Error {
                      }
                    }
                  }
                }
                n164 = case shown="No Error" w386 {
                  tunnel: [Station_Action."Wait Item In" Station_Action."ImformOut"] -> w385
                  frame No Error {
                  }
                  frame Error {
                  }
                }
              }
              frame 2 {
                w443 = T8[] [enum."S2站動作完成_29"] items=["S2站PC動作中_20", "電流量測完成產品OK_21", "電流量測完成產品NG_22", "S2站Format 執行_23", "S2 Format OK_24", "S2 Format NG_25", "S2站燒入執行_26", "S2站燒入OK_27", "S2站燒入NG_28", "S2站動作完成_29", "S3 PC動作中_30", "S3 Format 此站執行_31", "S3 Format OK_32", "S3 Format NG_33", "S3 燒入程式 此站執行_34", "S3 燒入程式 OK_35", "S3 燒入程式 NG_36", "S3 備用_37", "S3 備用_38", "S3 動作完成_39", "S4 PC動作中_40", "S4 量測完成 產品正常_41", "S4 量測完成 產品NG_42", "S4 Format 此站執行_43", "S4 Format OK_44", "S4 Format NG_45", "S4 燒入 此站不執行_46", "S4 燒入程式 OK_47", "S4 燒入程式 NG_48", "S4 藍芽Scan OK_49", "S4 藍芽Scan NG_50", "S4 動作完成_51", "給PLC要量電流訊號", "給PLC要量電壓訊號"]
                n165 = Add(x=w443, y=20) -> (x+y=w451:i32[])
                n166 = for {
                  tunnel: [w457] -> w450 mode=indexing
                  tunnel: w445 -> [w456]
                  tunnel: w451 -> [w455] mode=indexing
                  tunnel: bool[] [TRUE] ("Sat Coils") -> [w454]
                  n167 = Wait (ms)(milliseconds to wait=100) -> ()  [unwired: 1 out]
                  n168 = Bundle(cluster=T4 {"starting address"=0, "number of inputs"=0, "Sat Coils"=[], "Holding Registers"=[]} ("data"), "starting address"=w455, "number of inputs"=u16 0, "Sat Coils"=w454) -> (w460:T4)  [unwired: 1 in]
                  n169 = call "ModbusCmdIn.vi"("error in (no error)"=w456, "data"=w460, "Enum"=ModbusCmd."Set Coils") -> ("error out"=w457:errorcluster)  [unwired: 8 in]
                }
                n170 = Merge Errors(w450) -> (w449:errorcluster)
                n171 = while {
                  tunnel: w442 -> [w493]
                  tunnel: w441 -> [w492]
                  tunnel: [w485] -> w448
                  tunnel: [w488] -> w447
                  tunnel: w449 -> [w482]
                  stop <- w489 stop-if-true
                  n172 = property class="Bool (strict)"(reference=w492) -> ("Value"=w491:bool)  [unwired: 1 in, 2 out]
                  n173 = Not(x=w491) -> (.not. x?=w490:bool)
                  n174 = call "INWait_Name.vi"("FlowCtrl in"=w493, "Input2"=Auto_Inspection_IN_Name2."S2 Tool Format", "Wait?"=FALSE, "error in (no error)"=w482) -> ("StatusOut"=w487:bool, "error out"=w488:errorcluster)  [unwired: 8 in, 2 out]
                  n175 = Equal?(x=FALSE, y=w487) -> (x = y?=w485:bool)
                  n176 = Compound Arithmetic op=OR(w482, w485, w490) -> (w489:bool)
                  n177 = Wait (ms)(milliseconds to wait=123) -> ()  [unwired: 1 out]
                }
                n178 = case shown="True" w448 {
                  tunnel: w447 -> [w463 w469]
                  tunnel: [w463 w464] -> w440
                  frame False {
                  }
                  frame True {
                    w465 = T8[] [enum."S2站PC動作中_20", enum."電流量測完成產品OK_21", enum."電流量測完成產品NG_22", enum."S2站Format 執行_23", enum."S2 Format OK_24", enum."S2 Format NG_25", enum."S2站燒入執行_26", enum."S2站燒入OK_27", enum."S2站燒入NG_28", enum."S2站動作完成_29", enum."給PLC要量電流訊號"] items=["S2站PC動作中_20", "電流量測完成產品OK_21", "電流量測完成產品NG_22", "S2站Format 執行_23", "S2 Format OK_24", "S2 Format NG_25", "S2站燒入執行_26", "S2站燒入OK_27", "S2站燒入NG_28", "S2站動作完成_29", "S3 PC動作中_30", "S3 Format 此站執行_31", "S3 Format OK_32", "S3 Format NG_33", "S3 燒入程式 此站執行_34", "S3 燒入程式 OK_35", "S3 燒入程式 NG_36", "S3 備用_37", "S3 備用_38", "S3 動作完成_39", "S4 PC動作中_40", "S4 量測完成 產品正常_41", "S4 量測完成 產品NG_42", "S4 Format 此站執行_43", "S4 Format OK_44", "S4 Format NG_45", "S4 燒入 此站不執行_46", "S4 燒入程式 OK_47", "S4 燒入程式 NG_48", "S4 藍芽Scan OK_49", "S4 藍芽Scan NG_50", "S4 動作完成_51", "給PLC要量電流訊號", "給PLC要量電壓訊號"]
                    n179 = Add(x=w465, y=20) -> (x+y=w468:i32[])
                    n180 = for {
                      tunnel: w468 -> [w473] mode=indexing
                      tunnel: [w475] -> w470 mode=indexing
                      tunnel: w469 -> [w474]
                      n181 = Wait (ms)(milliseconds to wait=100) -> ()  [unwired: 1 out]
                      n182 = Bundle(cluster=T4 {"starting address"=0, "number of inputs"=0, "Sat Coils"=[], "Holding Registers"=[]} ("data"), "starting address"=w473, "number of inputs"=u16 0, "Sat Coils"=bool[] [FALSE]) -> (w478:T4)  [unwired: 1 in]
                      n183 = call "ModbusCmdIn.vi"("error in (no error)"=w474, "data"=w478, "Enum"=ModbusCmd."Set Coils") -> ("error out"=w475:errorcluster)  [unwired: 8 in]
                    }
                    n184 = Merge Errors(w470) -> (w467:errorcluster)
                    n185 = case shown="No Error" w467 {
                      selector: w467 -> [w471 w472]
                      tunnel: [w471 w472] -> w464
                      frame No Error {
                      }
                      frame Error {
                      }
                    }
                  }
                }
                n186 = case shown="No Error" w440 {
                  tunnel: [Station_Action."Wait Item In" Station_Action."ImformOut"] -> w439
                  frame No Error {
                  }
                  frame Error {
                  }
                }
              }
              frame 3 {
                w500 = T8[] [enum."S3 動作完成_39"] items=["S2站PC動作中_20", "電流量測完成產品OK_21", "電流量測完成產品NG_22", "S2站Format 執行_23", "S2 Format OK_24", "S2 Format NG_25", "S2站燒入執行_26", "S2站燒入OK_27", "S2站燒入NG_28", "S2站動作完成_29", "S3 PC動作中_30", "S3 Format 此站執行_31", "S3 Format OK_32", "S3 Format NG_33", "S3 燒入程式 此站執行_34", "S3 燒入程式 OK_35", "S3 燒入程式 NG_36", "S3 備用_37", "S3 備用_38", "S3 動作完成_39", "S4 PC動作中_40", "S4 量測完成 產品正常_41", "S4 量測完成 產品NG_42", "S4 Format 此站執行_43", "S4 Format OK_44", "S4 Format NG_45", "S4 燒入 此站不執行_46", "S4 燒入程式 OK_47", "S4 燒入程式 NG_48", "S4 藍芽Scan OK_49", "S4 藍芽Scan NG_50", "S4 動作完成_51", "給PLC要量電流訊號", "給PLC要量電壓訊號"]
                n187 = Add(x=w500, y=20) -> (x+y=w508:i32[])
                n188 = for {
                  tunnel: [w514] -> w507 mode=indexing
                  tunnel: w502 -> [w513]
                  tunnel: w508 -> [w512] mode=indexing
                  tunnel: bool[] [TRUE] ("Sat Coils") -> [w511]
                  n189 = Wait (ms)(milliseconds to wait=100) -> ()  [unwired: 1 out]
                  n190 = Bundle(cluster=T4 {"starting address"=0, "number of inputs"=0, "Sat Coils"=[], "Holding Registers"=[]} ("data"), "starting address"=w512, "number of inputs"=u16 0, "Sat Coils"=w511) -> (w517:T4)  [unwired: 1 in]
                  n191 = call "ModbusCmdIn.vi"("error in (no error)"=w513, "data"=w517, "Enum"=ModbusCmd."Set Coils") -> ("error out"=w514:errorcluster)  [unwired: 8 in]
                }
                n192 = Merge Errors(w507) -> (w506:errorcluster)
                n193 = while {
                  tunnel: w499 -> [w550]
                  tunnel: w498 -> [w549]
                  tunnel: [w542] -> w505
                  tunnel: [w545] -> w504
                  tunnel: w506 -> [w539]
                  stop <- w546 stop-if-true
                  n194 = property class="Bool (strict)"(reference=w549) -> ("Value"=w548:bool)  [unwired: 1 in, 2 out]
                  n195 = Not(x=w548) -> (.not. x?=w547:bool)
                  n196 = call "INWait_Name.vi"("FlowCtrl in"=w550, "Input2"=Auto_Inspection_IN_Name2."S3 Tool Prpgram", "Wait?"=FALSE, "error in (no error)"=w539) -> ("StatusOut"=w544:bool, "error out"=w545:errorcluster)  [unwired: 8 in, 2 out]
                  n197 = Equal?(x=FALSE, y=w544) -> (x = y?=w542:bool)
                  n198 = Compound Arithmetic op=OR(w539, w542, w547) -> (w546:bool)
                  n199 = Wait (ms)(milliseconds to wait=123) -> ()  [unwired: 1 out]
                }
                n200 = case shown="True" w505 {
                  tunnel: w504 -> [w520 w526]
                  tunnel: [w520 w523] -> w495
                  tunnel: w497 -> [_ _]
                  frame False {
                  }
                  frame True {
                    w521 = T8[] [enum."S3 PC動作中_30", enum."S3 Format OK_32", enum."S3 Format NG_33", enum."S3 燒入程式 OK_35", enum."S3 燒入程式 NG_36", enum."S3 動作完成_39"] items=["S2站PC動作中_20", "電流量測完成產品OK_21", "電流量測完成產品NG_22", "S2站Format 執行_23", "S2 Format OK_24", "S2 Format NG_25", "S2站燒入執行_26", "S2站燒入OK_27", "S2站燒入NG_28", "S2站動作完成_29", "S3 PC動作中_30", "S3 Format 此站執行_31", "S3 Format OK_32", "S3 Format NG_33", "S3 燒入程式 此站執行_34", "S3 燒入程式 OK_35", "S3 燒入程式 NG_36", "S3 備用_37", "S3 備用_38", "S3 動作完成_39", "S4 PC動作中_40", "S4 量測完成 產品正常_41", "S4 量測完成 產品NG_42", "S4 Format 此站執行_43", "S4 Format OK_44", "S4 Format NG_45", "S4 燒入 此站不執行_46", "S4 燒入程式 OK_47", "S4 燒入程式 NG_48", "S4 藍芽Scan OK_49", "S4 藍芽Scan NG_50", "S4 動作完成_51", "給PLC要量電流訊號", "給PLC要量電壓訊號"]
                    n201 = Add(x=w521, y=20) -> (x+y=w525:i32[])
                    n202 = for {
                      tunnel: w525 -> [w530] mode=indexing
                      tunnel: [w532] -> w527 mode=indexing
                      tunnel: w526 -> [w531]
                      n203 = Wait (ms)(milliseconds to wait=100) -> ()  [unwired: 1 out]
                      n204 = Bundle(cluster=T4 {"starting address"=0, "number of inputs"=0, "Sat Coils"=[], "Holding Registers"=[]} ("data"), "starting address"=w530, "number of inputs"=u16 0, "Sat Coils"=bool[] [FALSE]) -> (w535:T4)  [unwired: 1 in]
                      n205 = call "ModbusCmdIn.vi"("error in (no error)"=w531, "data"=w535, "Enum"=ModbusCmd."Set Coils") -> ("error out"=w532:errorcluster)  [unwired: 8 in]
                    }
                    n206 = Merge Errors(w527) -> (w524:errorcluster)
                    n207 = case shown="Error .." w524 {
                      selector: w524 -> [w528 w529]
                      tunnel: [w528 w529] -> w523
                      frame No Error {
                      }
                      frame Error {
                      }
                    }
                  }
                }
                n208 = case shown="No Error" w495 {
                  tunnel: [Station_Action."Wait Item In" Station_Action."ImformOut"] -> w496
                  frame No Error {
                  }
                  frame Error {
                  }
                }
              }
              frame 4 {
                w552 = T8[] [enum."S4 動作完成_51"] items=["S2站PC動作中_20", "電流量測完成產品OK_21", "電流量測完成產品NG_22", "S2站Format 執行_23", "S2 Format OK_24", "S2 Format NG_25", "S2站燒入執行_26", "S2站燒入OK_27", "S2站燒入NG_28", "S2站動作完成_29", "S3 PC動作中_30", "S3 Format 此站執行_31", "S3 Format OK_32", "S3 Format NG_33", "S3 燒入程式 此站執行_34", "S3 燒入程式 OK_35", "S3 燒入程式 NG_36", "S3 備用_37", "S3 備用_38", "S3 動作完成_39", "S4 PC動作中_40", "S4 量測完成 產品正常_41", "S4 量測完成 產品NG_42", "S4 Format 此站執行_43", "S4 Format OK_44", "S4 Format NG_45", "S4 燒入 此站不執行_46", "S4 燒入程式 OK_47", "S4 燒入程式 NG_48", "S4 藍芽Scan OK_49", "S4 藍芽Scan NG_50", "S4 動作完成_51", "給PLC要量電流訊號", "給PLC要量電壓訊號"]
                n209 = Add(x=w552, y=20) -> (x+y=w564:i32[])
                n210 = for {
                  tunnel: [w570] -> w563 mode=indexing
                  tunnel: w556 -> [w569]
                  tunnel: w564 -> [w568] mode=indexing
                  tunnel: bool[] [TRUE] ("Sat Coils") -> [w567]
                  n211 = Wait (ms)(milliseconds to wait=100) -> ()  [unwired: 1 out]
                  n212 = Bundle(cluster=T4 {"starting address"=0, "number of inputs"=0, "Sat Coils"=[], "Holding Registers"=[]} ("data"), "starting address"=w568, "number of inputs"=u16 0, "Sat Coils"=w567) -> (w573:T4)  [unwired: 1 in]
                  n213 = call "ModbusCmdIn.vi"("error in (no error)"=w569, "data"=w573, "Enum"=ModbusCmd."Set Coils") -> ("error out"=w570:errorcluster)  [unwired: 8 in]
                }
                n214 = Merge Errors(w563) -> (w562:errorcluster)
                n215 = while {
                  tunnel: w555 -> [w618]
                  tunnel: w554 -> [w617]
                  tunnel: [w610] -> w561
                  tunnel: [w613] -> w560
                  tunnel: w562 -> [w607]
                  stop <- w614 stop-if-true
                  n216 = property class="Bool (strict)"(reference=w617) -> ("Value"=w616:bool)  [unwired: 1 in, 2 out]
                  n217 = Not(x=w616) -> (.not. x?=w615:bool)
                  n218 = call "INWait_Name.vi"("FlowCtrl in"=w618, "Input2"=Auto_Inspection_IN_Name2."S4 Tool Sacn", "Wait?"=FALSE, "error in (no error)"=w607) -> ("StatusOut"=w612:bool, "error out"=w613:errorcluster)  [unwired: 8 in, 2 out]
                  n219 = Equal?(x=FALSE, y=w612) -> (x = y?=w610:bool)
                  n220 = Compound Arithmetic op=OR(w607, w610, w615) -> (w614:bool)
                  n221 = Wait (ms)(milliseconds to wait=123) -> ()  [unwired: 1 out]
                }
                n222 = case shown="True" w561 {
                  tunnel: w560 -> [w576 w582]
                  tunnel: [w576 w579] -> w558
                  frame False {
                  }
                  frame True {
                    w577 = T8[] [enum."S4 PC動作中_40", enum."S4 量測完成 產品正常_41", enum."S4 量測完成 產品NG_42", enum."S4 Format OK_44", enum."S4 Format NG_45", enum."S4 燒入程式 OK_47", enum."S4 燒入程式 NG_48", enum."S4 藍芽Scan OK_49", enum."S4 藍芽Scan NG_50", enum."S4 動作完成_51", enum."給PLC要量電壓訊號"] items=["S2站PC動作中_20", "電流量測完成產品OK_21", "電流量測完成產品NG_22", "S2站Format 執行_23", "S2 Format OK_24", "S2 Format NG_25", "S2站燒入執行_26", "S2站燒入OK_27", "S2站燒入NG_28", "S2站動作完成_29", "S3 PC動作中_30", "S3 Format 此站執行_31", "S3 Format OK_32", "S3 Format NG_33", "S3 燒入程式 此站執行_34", "S3 燒入程式 OK_35", "S3 燒入程式 NG_36", "S3 備用_37", "S3 備用_38", "S3 動作完成_39", "S4 PC動作中_40", "S4 量測完成 產品正常_41", "S4 量測完成 產品NG_42", "S4 Format 此站執行_43", "S4 Format OK_44", "S4 Format NG_45", "S4 燒入 此站不執行_46", "S4 燒入程式 OK_47", "S4 燒入程式 NG_48", "S4 藍芽Scan OK_49", "S4 藍芽Scan NG_50", "S4 動作完成_51", "給PLC要量電流訊號", "給PLC要量電壓訊號"]
                    n223 = Add(x=w577, y=20) -> (x+y=w581:i32[])
                    n224 = for {
                      tunnel: w581 -> [w598] mode=indexing
                      tunnel: [w600] -> w583 mode=indexing
                      tunnel: w582 -> [w599]
                      n225 = Wait (ms)(milliseconds to wait=100) -> ()  [unwired: 1 out]
                      n226 = Bundle(cluster=T4 {"starting address"=0, "number of inputs"=0, "Sat Coils"=[], "Holding Registers"=[]} ("data"), "starting address"=w598, "number of inputs"=u16 0, "Sat Coils"=bool[] [FALSE]) -> (w603:T4)  [unwired: 1 in]
                      n227 = call "ModbusCmdIn.vi"("error in (no error)"=w599, "data"=w603, "Enum"=ModbusCmd."Set Coils") -> ("error out"=w600:errorcluster)  [unwired: 8 in]
                    }
                    n228 = Merge Errors(w583) -> (w580:errorcluster)
                    n229 = case shown="No Error" w580 {
                      selector: w580 -> [w584 w597]
                      tunnel: [w585 w597] -> w579
                      frame No Error {
                        n230 = disable-structure shown="Disabled" {
                          disable-tunnel: [w594 _] -> w585
                          disable-tunnel: w584 -> [w593 _]
                          frame Disabled {
                            # "收尋S4站條碼"
                            n231 = global read "Main Glb.vi" "Input Registers0-99"() -> (w592:u16[])
                            n232 = call "Red PLC InReg.vi"("length"=10, "index"=40, "Input Registers Arr"=w592) -> ("Rad In Reg"=w591:string)  [unwired: 7 in, 1 out]
                            n233 = call "Table Sav and Del.vi"("error in (no error)"=w593, "SN"=w591) -> ("error out"=w587:errorcluster, "未找到條碼"=w588:bool)  [unwired: 8 in]
                            n234 = case shown="True" w588 {
                              tunnel: [_ w595] -> w586
                              frame False {
                              }
                              frame True {
                                n235 = disable-structure shown="Disabled" {
                                disable-tunnel: [errorcluster {"status"=TRUE, "code"=18407, "source"=""} ("error in (no error)") _] -> w595
                                frame Disabled {
                                }
                                frame Enabled {
                                }
                                }
                              }
                            }
                            n236 = Merge Errors(w587, w586) -> (w594:errorcluster)
                          }
                          frame Enabled {
                          }
                        }
                      }
                      frame Error {
                      }
                    }
                  }
                }
                n237 = case shown="No Error" w558 {
                  tunnel: [Station_Action."Wait Item In" Station_Action."ImformOut"] -> w557
                  frame No Error {
                  }
                  frame Error {
                  }
                }
              }
              frame 5 {
                w620 = T9[] [enum."S11雷射測高完成"] items=["S11雷射測量動作中", "S11雷射測點1完成", "S11雷射測點2完成", "S11雷測測量OK", "S11雷測測量NG", "S11雷測測量重測", "S11備用_6", "S11備用_7", "S11備用_8", "S11雷射測高完成"]
                n238 = Add(x=w620, y=110) -> (x+y=w632:i32[])
                n239 = for {
                  tunnel: [w638] -> w631 mode=indexing
                  tunnel: w626 -> [w637]
                  tunnel: w632 -> [w636] mode=indexing
                  tunnel: bool[] [TRUE] ("Sat Coils") -> [w635]
                  n240 = Wait (ms)(milliseconds to wait=100) -> ()  [unwired: 1 out]
                  n241 = Bundle(cluster=T4 {"starting address"=0, "number of inputs"=0, "Sat Coils"=[], "Holding Registers"=[]} ("data"), "starting address"=w636, "number of inputs"=u16 0, "Sat Coils"=w635) -> (w641:T4)  [unwired: 1 in]
                  n242 = call "ModbusCmdIn.vi"("error in (no error)"=w637, "data"=w641, "Enum"=ModbusCmd."Set Coils") -> ("error out"=w638:errorcluster)  [unwired: 8 in]
                }
                n243 = Merge Errors(w631) -> (w630:errorcluster)
                n244 = while {
                  tunnel: w625 -> [w674]
                  tunnel: w624 -> [w673]
                  tunnel: [w666] -> w629
                  tunnel: [w669] -> w628
                  tunnel: w630 -> [w663]
                  stop <- w670 stop-if-true
                  n245 = property class="Bool (strict)"(reference=w673) -> ("Value"=w672:bool)  [unwired: 1 in, 2 out]
                  n246 = Not(x=w672) -> (.not. x?=w671:bool)
                  n247 = call "INWait_Name.vi"("FlowCtrl in"=w674, "Input2"=Auto_Inspection_IN_Name2."S11 Laser Detect", "Wait?"=FALSE, "error in (no error)"=w663) -> ("StatusOut"=w668:bool, "error out"=w669:errorcluster)  [unwired: 8 in, 2 out]
                  n248 = Equal?(x=FALSE, y=w668) -> (x = y?=w666:bool)
                  n249 = Compound Arithmetic op=OR(w663, w666, w671) -> (w670:bool)
                  n250 = Wait (ms)(milliseconds to wait=123) -> ()  [unwired: 1 out]
                }
                n251 = case shown="True" w629 {
                  tunnel: w628 -> [w644 w650]
                  tunnel: [w644 w647] -> w622
                  frame False {
                  }
                  frame True {
                    w645 = T9[] [enum."S11雷射測量動作中", enum."S11雷射測點1完成", enum."S11雷射測點2完成", enum."S11雷測測量OK", enum."S11雷測測量NG", enum."S11雷測測量重測", enum."S11雷射測高完成"] items=["S11雷射測量動作中", "S11雷射測點1完成", "S11雷射測點2完成", "S11雷測測量OK", "S11雷測測量NG", "S11雷測測量重測", "S11備用_6", "S11備用_7", "S11備用_8", "S11雷射測高完成"]
                    n252 = Add(x=w645, y=110) -> (x+y=w649:i32[])
                    n253 = for {
                      tunnel: w649 -> [w654] mode=indexing
                      tunnel: [w656] -> w651 mode=indexing
                      tunnel: w650 -> [w655]
                      n254 = Wait (ms)(milliseconds to wait=100) -> ()  [unwired: 1 out]
                      n255 = Bundle(cluster=T4 {"starting address"=0, "number of inputs"=0, "Sat Coils"=[], "Holding Registers"=[]} ("data"), "starting address"=w654, "number of inputs"=u16 0, "Sat Coils"=bool[] [FALSE]) -> (w659:T4)  [unwired: 1 in]
                      n256 = call "ModbusCmdIn.vi"("error in (no error)"=w655, "data"=w659, "Enum"=ModbusCmd."Set Coils") -> ("error out"=w656:errorcluster)  [unwired: 8 in]
                    }
                    n257 = Merge Errors(w651) -> (w648:errorcluster)
                    n258 = case shown="No Error" w648 {
                      selector: w648 -> [w652 w653]
                      tunnel: [w652 w653] -> w647
                      frame No Error {
                      }
                      frame Error {
                      }
                    }
                  }
                }
                n259 = case shown="Error .." w622 {
                  tunnel: [Station_Action."Wait Item In" Station_Action."ImformOut"] -> w623
                  frame No Error {
                  }
                  frame Error {
                  }
                }
              }
            }
          }
        }
        n260 = Number To Decimal String(number=w36) -> (decimal integer string=w37:string)  [unwired: 1 in]
        n261 = call-dynamic "Write FGV Data.vi"("Station Action in"=w35, "0Cv/1St"=1, "DataIn"=w37) -> ("Station Action out"=w34:refnum<class "Station Action.lvclass">)  [unwired: 11 in, 1 out]
        n262 = case shown="Error .." w33 {
          selector: w33 -> [_ w72]
          tunnel: w34 -> [_ w71]
          frame No Error {
          }
          frame Error {
            w66 = Auto_Inspection_Data_Name."LocalRun" ("Data")
            w63 = "0" ("DataIn")
            n263 = call-dynamic "WriteFGVError.vi"("error in (no error)"=w72, "0Cv/1St"=1, "Station Action in"=w71) -> ("error out"=w64:errorcluster, "Station Action out"=w67:refnum<class "Station Action.lvclass">)  [unwired: 7 in]
            n264 = call-dynamic "Write FGV Data.vi"("Station Action in"=w67, "0Cv/1St"=0, "DataIn"=w63, "Data"=w66, "error in (no error)"=w64) -> ("Station Action out"=w68:refnum<class "Station Action.lvclass">, "error out"=w65:errorcluster)  [unwired: 9 in]
            n265 = call-dynamic "Write FGV Data.vi"("Station Action in"=w68, "0Cv/1St"=1, "DataIn"=w63, "Data"=w66, "error in (no error)"=w65) -> ("error out"=w62:errorcluster)  [unwired: 9 in, 1 out]
            n266 = call <vilib>:"Clear Errors.vi"("error in (no error)"=w62) -> ()  [unwired: 5 in, 2 out]
          }
        }
        n267 = case shown="Error .." w33 {
          frame No Error {
          }
          frame Error {
            # "PC Alarm"
            # "PC-->PLC  PC Auto"
            n268 = Bundle(cluster=T4 {"starting address"=0, "number of inputs"=0, "Sat Coils"=[], "Holding Registers"=[]} ("data"), "starting address"=6, "number of inputs"=u16 0, "Sat Coils"=bool[] [TRUE]) -> (w55:T4)  [unwired: 1 in]
            n269 = Bundle(cluster=T4 {"starting address"=0, "number of inputs"=0, "Sat Coils"=[], "Holding Registers"=[]} ("data"), "starting address"=1, "number of inputs"=u16 0, "Sat Coils"=bool[] [FALSE]) -> (w56:T4)  [unwired: 1 in]
            n270 = call "ModbusCmdIn.vi"("data"=w56, "Enum"=ModbusCmd."Set Coils") -> ("error out"=w49:errorcluster)  [unwired: 9 in]
            n271 = call "ModbusCmdIn.vi"("error in (no error)"=w49, "data"=w55, "Enum"=ModbusCmd."Set Coils") -> ("error out"=w48:errorcluster)  [unwired: 8 in]
            n272 = call <vilib>:"Clear Errors.vi"("error in (no error)"=w48) -> ()  [unwired: 5 in, 2 out]
          }
        }
        n273 = property class="Enum (strict)"(reference=w44, "Value"=w36) -> ()  [unwired: 1 in, 2 out]
      }
    }
    n274 = call "Exit.vi"() -> ("ExitOut"=w19:bool)  [unwired: 11 in]
  }
  n275 = disable-structure shown="Disabled" {
    frame Disabled {
      n276 = case shown="0, Default" {
        selector: _ -> [_ _ _ _ _ _]
        tunnel: [Auto_Inspection_IN_Name2."S0 Station" Auto_Inspection_IN_Name2."S1 Barcode " Auto_Inspection_IN_Name2."S2 Tool Format" Auto_Inspection_IN_Name2."S3 Tool Prpgram" Auto_Inspection_IN_Name2."S4 Tool Sacn" Auto_Inspection_IN_Name2."S11 Laser Detect"] -> w676
        frame 0, Default {
        }
        frame 1 {
        }
        frame 2 {
        }
        frame 3 {
        }
        frame 4 {
        }
        frame 5 {
        }
      }
      n277 = call "INWait_Name.vi"("Input2"=w676) -> ()  [unwired: 11 in, 4 out]
    }
    frame Enabled {
    }
  }
  n278 = disable-structure shown="Disabled" {
    disable-tunnel: _ -> [w683 _]
    frame Disabled {
      n279 = call "Auto Inspection_Status.vi"("Action"=enum16{"Initial", "Write", "Read"}."Write", "DataIn"="wait input", "Station"=Auto_Inspection_Station_Name2."S1Barcode", "Data"=Auto_Inspection_Data_Name."CurrentAction", "error in"=w683) -> ()  [unwired: 8 in, 3 out]
    }
    frame Enabled {
    }
  }
  n280 = disable-structure shown="Disabled" {
    frame Disabled {
      n281 = flat-sequence {
        tunnel: _ -> [w702]
        tunnel: _ -> [w700]
        frame #0 {
          n282 = Variant To Data(type=T11 {"LineScan arrive"=refnum, "LineScanfinish"=refnum, "AI arrive"=refnum, "AI finish"=refnum, "NG Pick arrive"=refnum, "NG Pick finish"=refnum} ("UI Ref"), Variant=w700) -> (data=w692:T11)  [unwired: 1 in, 1 out]
          n283 = call-dynamic "Read UIRef.vi"("0Arrive/1Finish"=1, "UI Ref"=w692, "Station Action in"=w702) -> ("error out"=w695:errorcluster, "RefOut"=w701:refnum<vi>, "Station Action out"=w696:refnum<class "Station Action.lvclass">)  [unwired: 6 in]
          n284 = property class="Bool (strict)"(reference=w701, error in=w695, "Value"=TRUE) -> (reference out=w689:refnum<vi>, error out=w694:errorcluster)
          n285 = call-dynamic "Read UIRef.vi"("error in (no error)"=w694, "0Arrive/1Finish"=0, "UI Ref"=w692, "Station Action in"=w696) -> ("RefOut"=w691:refnum<vi>)  [unwired: 5 in, 2 out]
          n286 = while {
            tunnel: w691 -> [w708]
            tunnel: [w703] -> w688
            stop <- w707 stop-if-true
            n287 = property on="Property Node" class="Bool (strict)"(reference=w708) -> (error out=w703:errorcluster, "Value"=w706:bool)  [unwired: 1 in, 1 out]
            n288 = Wait (ms)(milliseconds to wait=u32 33) -> ()  [unwired: 1 out]
            n289 = Equal?(x=w706, y=FALSE) -> (x = y?=w707:bool)
          }
          n290 = property class="Bool (strict)"(reference=w689, error in=w688, "Value"=FALSE) -> ()  [unwired: 2 out]
        }
      }
    }
    frame Enabled {
    }
  }
